vi "Main.vi"(0 "A":dbl=5.0, 5 "B":dbl=7.0, 7 "Calculate":bool, 11 "error in":errorcluster, 13 "Operations":T1) -> (4 "C":dbl, 15 "error out":errorcluster)   [LabVIEW 2023]
doc: "This is a simple calculator which can perform basic arithmetic operations like add, subtract, multiply and divide."
uses:
  Typedef/Operations.ctl
  Typedef/ClassClusters.ctl
  Arithmetic/Arithmetic.lvclass
  Typedef/QueueOperations.ctl
  Children/Multiply/Multiply.lvclass
  Children/Add/Add.lvclass
  Children/Divide/Divide.lvclass
panel:
  # "CALCULATOR"
  # "DISPLAY"
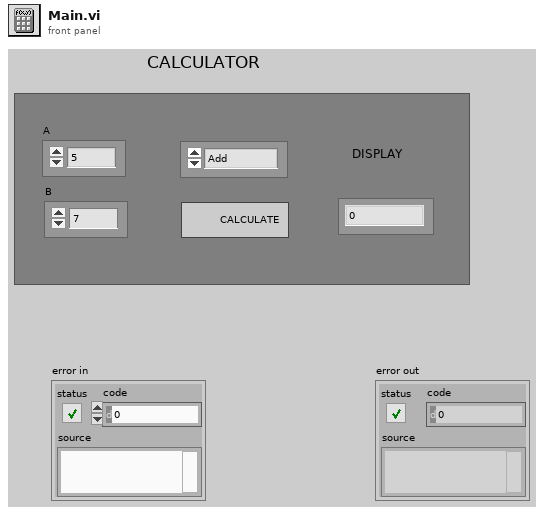
[diagram p1: front panel]
types:
  T1 = typedef "Operations.ctl" = enum16{"Add", "Subtract", "Multiply", "Divide"}
  T2 = typedef "QueueOperations.ctl" = enum16{"Create", "Enqueue", "Enqueue N elements", "Dequeue", "Flush", "Release"}
  T3 = typedef "ClassClusters.ctl" = cluster{"A":dbl, "B":dbl, "C":dbl, "generic class reference":refnum<class "Arithmetic.lvclass">, "Check":bool, "Operations":T1, "Parent Class":refnum<class "Arithmetic.lvclass">, "Add ":refnum<class "Arithmetic.lvclass">, "Subtract":refnum<class "Arithmetic.lvclass">, "Multiply":refnum<class "Arithmetic.lvclass">, "Divide":refnum<class "Arithmetic.lvclass">}
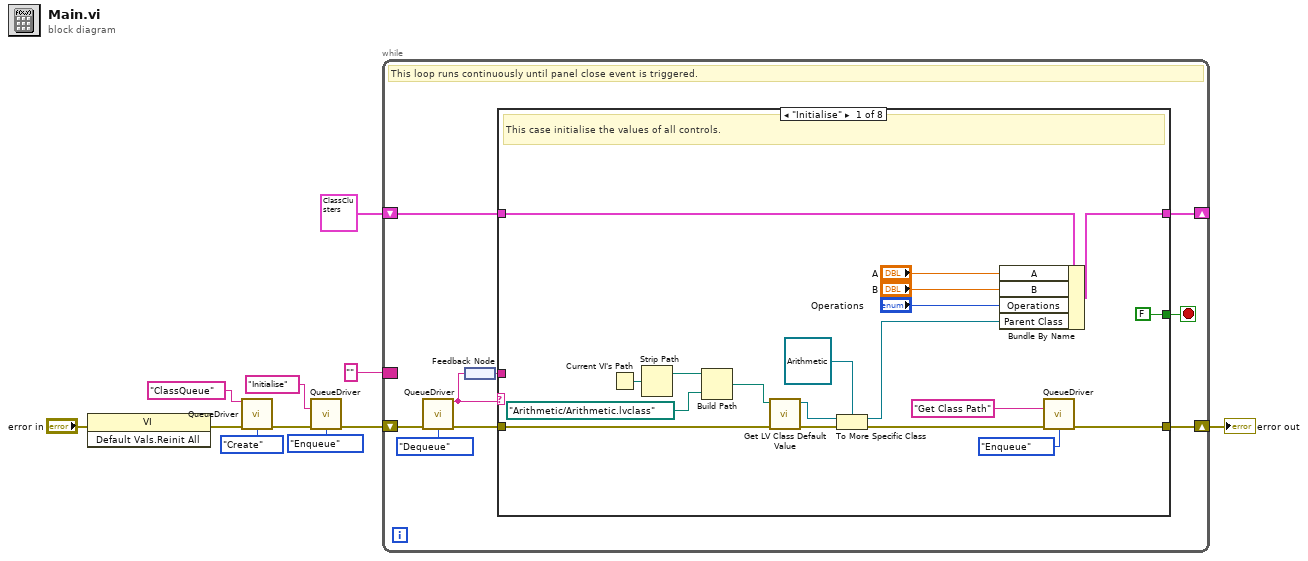
[diagram p0: block diagram]
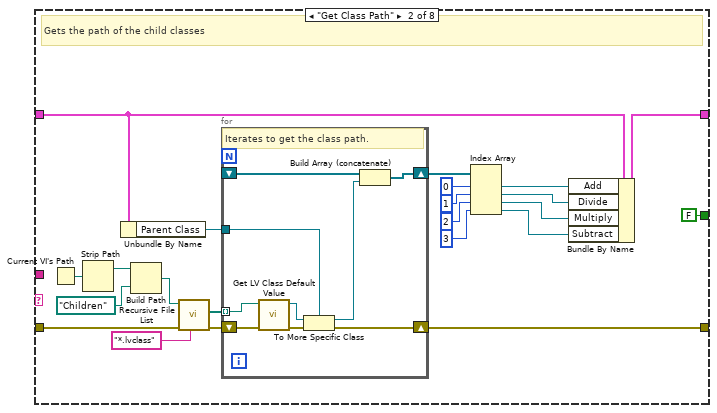
[diagram p2: hidden frame]
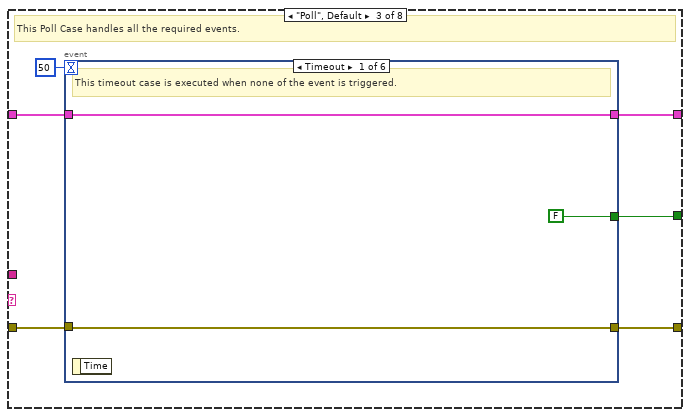
[diagram p3: hidden frame]
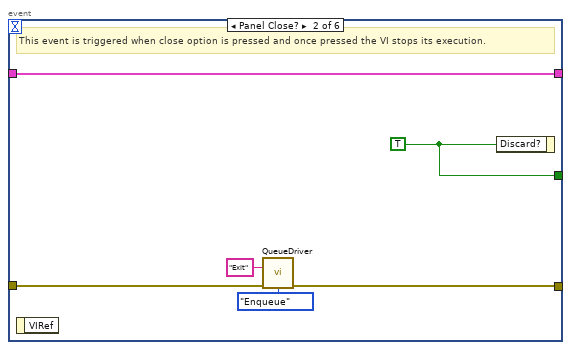
[diagram p4: hidden frame]
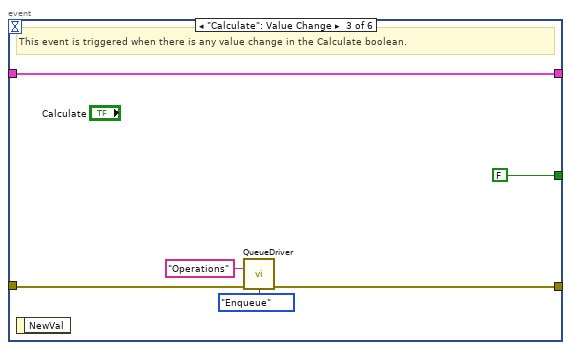
[diagram p5: hidden frame]
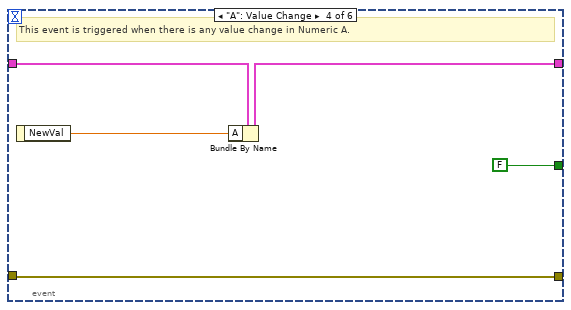
[diagram p6: hidden frame]
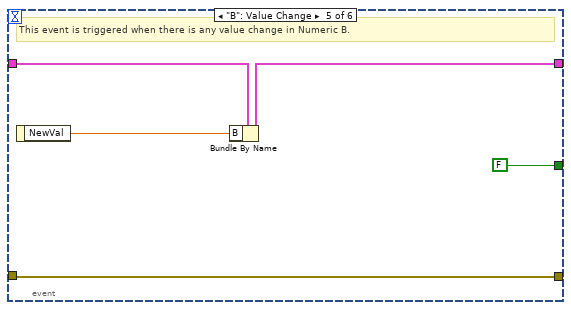
[diagram p7: hidden frame]
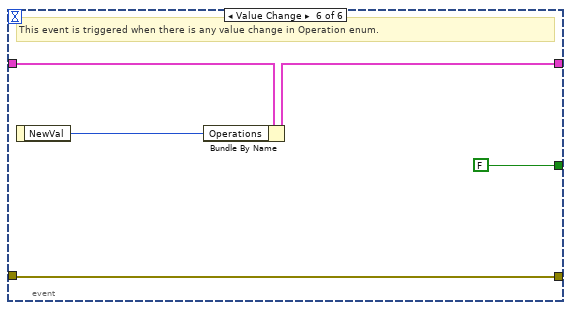
[diagram p8: hidden frame]
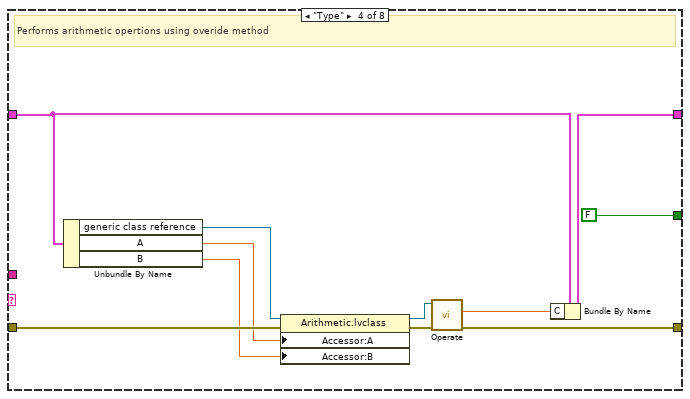
[diagram p9: hidden frame]
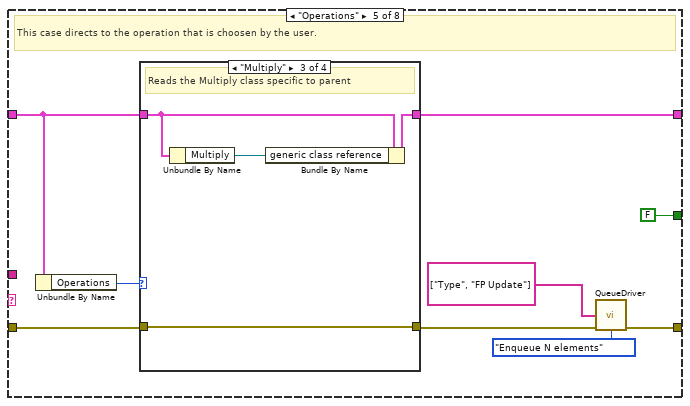
[diagram p10: hidden frame]
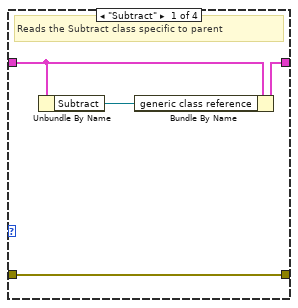
[diagram p11: hidden frame]
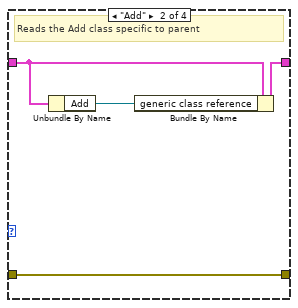
[diagram p12: hidden frame]
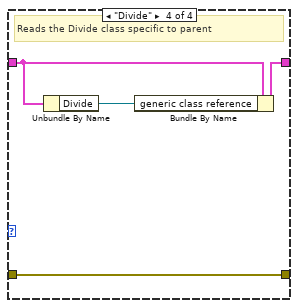
[diagram p13: hidden frame]
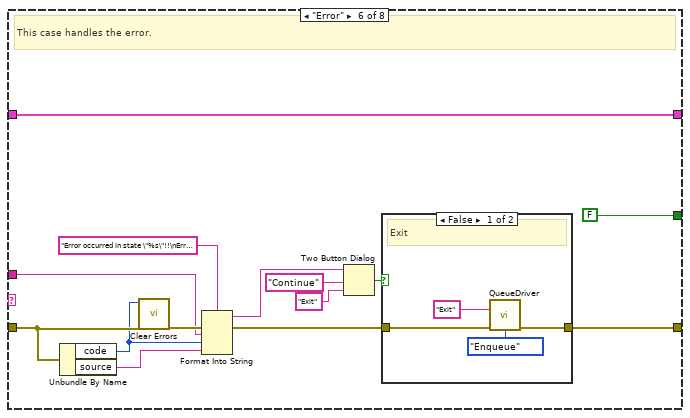
[diagram p14: hidden frame]
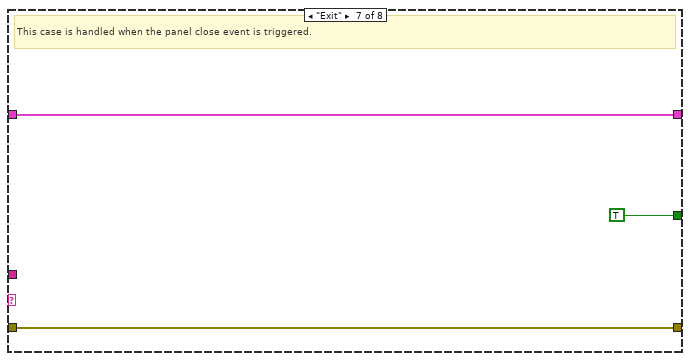
[diagram p16: hidden frame]
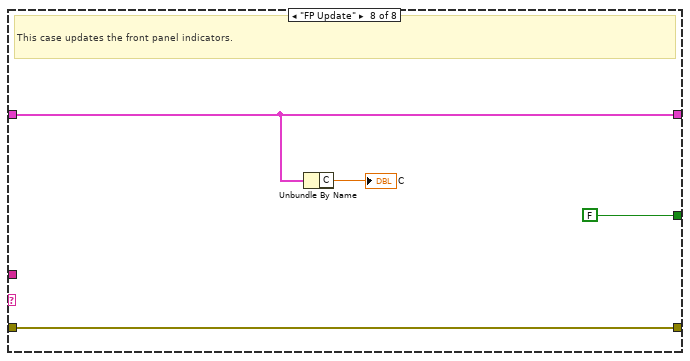
[diagram p17: hidden frame]
diagram:
  n1 = invoke class="VI" method="Default Vals.Reinit All"(error in="error in") -> (error out=w1:errorcluster)  [unwired: 2 in, 2 out]
  n2 = call "QueueDriver.vi"("Queue Name"="ClassQueue", "error in"=w1, "Queue Operations"=QueueOperations."Create") -> ("error out"=w10:errorcluster)  [unwired: 11 in, 1 out]
  n3 = call "QueueDriver.vi"("Enqueue State"="Initialise", "error in"=w10, "Queue Operations"=QueueOperations."Enqueue") -> ("error out"=w9:errorcluster)  [unwired: 11 in, 1 out]
  n4 = while {
    shift-right: [w19] -> _
    shift-left: T3 {"A"=0.0, "B"=0.0, "C"=0.0, "generic class reference"=refnum, "Check"=FALSE, "Operations"=enum."Add", "Parent Class"=refnum, "Add "=refnum, "Subtract"=refnum, "Multiply"=refnum, "Divide"=refnum} -> [w20]
    shift-right: [w15] -> w2
    shift-left: w9 -> [w18]
    border: "" ("Dequeue State") -> [_]
    stop <- w12 stop-if-true
    # "This loop runs continuously until panel close event is triggered."
    n5 = call "QueueDriver.vi"("error in"=w18, "Queue Operations"=QueueOperations."Dequeue") -> ("Dequeue State"=w14:string, "error out"=w17:errorcluster)  [unwired: 12 in]
    n6 = feedback-in #1(w14) -> ()
    n7 = feedback #1() -> (w13:string)
    n8 = case shown="\"Initialise\"" w14 {
      tunnel: w20 -> [w39 w41 w76 w117 w119 w156 w163 w167]
      tunnel: [w38 w46 w75 w110 w118 w156 w163 w167] -> w19
      tunnel: w17 -> [w33 w61 w72 w115 w125 w146 w164 w168]
      tunnel: [w22 w60 w74 w108 w122 w147 w164 w168] -> w15
      tunnel: w13 -> [_ _ _ _ _ w145 _ _]
      tunnel: [FALSE ("Check") FALSE ("Check") w71 FALSE ("Check") FALSE ("Check") FALSE ("Check") TRUE ("Check") FALSE ("Check")] -> w12
      frame "Initialise" {
        # "This case initialise the values of all controls."
        n9 = Current VI's Path() -> (path=w31:path)
        n10 = Strip Path(path=w31) -> (stripped path=w30:path)  [unwired: 1 out]
        n11 = Build Path(base path=w30, name or relative path=path "Arithmetic/Arithmetic.lvclass") -> (appended path=w28:path)
        n12 = call <vilib>:"Get LV Class Default Value.vi"("error in (no error)"=w33, "class path"=w28) -> ("error out"=w32:errorcluster, "object"=w27:refnum<class>)  [unwired: 8 in]
        n13 = To More Specific Class(target class=refnum<class "Arithmetic.lvclass"> refnum ("Arithmetic.lvclass"), reference=w27, error in=w32) -> (specific class reference=w25:refnum<class "Arithmetic.lvclass">, error out=w23:errorcluster)
        n14 = Bundle By Name(cluster=w39, "A"="A", "B"="B", "Operations"="Operations", "Parent Class"=w25) -> (w38:T3)
        n15 = call "QueueDriver.vi"("Enqueue State"="Get Class Path", "error in"=w23, "Queue Operations"=QueueOperations."Enqueue") -> ("error out"=w22:errorcluster)  [unwired: 11 in, 1 out]
      }
      frame "Get Class Path" {
        # "Gets the path of the child classes"
        n16 = Current VI's Path() -> (path=w58:path)
        n17 = Strip Path(path=w58) -> (stripped path=w57:path)  [unwired: 1 out]
        n18 = Unbundle By Name(w41) -> ("Parent Class"=w40:refnum<class "Arithmetic.lvclass">)
        n19 = Build Path(base path=w57, name or relative path=path "Children") -> (appended path=w54:path)
        n20 = call <vilib>:"Recursive File List.vi"("pattern"="*.lvclass", "error in (no error)"=w61, "Folder Path"=w54) -> ("error out"=w55:errorcluster, "All Files in Dir"=w52:path[])  [unwired: 4 in, 3 out]
        n21 = for {
          shift-right: [w65] -> w60
          shift-left: w55 -> [w70]
          shift-right: [w67] -> w51
          shift-left: _ -> [w66]
          tunnel: w52 -> [w69] mode=indexing
          tunnel: w40 -> [w62]
          # "Iterates to get the class path."
          n22 = call <vilib>:"Get LV Class Default Value.vi"("error in (no error)"=w70, "class path"=w69) -> ("error out"=w68:errorcluster, "object"=w64:refnum<class>)  [unwired: 8 in]
          n23 = To More Specific Class(target class=w62, reference=w64, error in=w68) -> (specific class reference=w63:refnum<class "Arithmetic.lvclass">, error out=w65:errorcluster)
          n24 = Build Array (concatenate)(w66, w63) -> (w67:refnum<class "Arithmetic.lvclass">[])
        }
        n25 = Index Array(array=w51, index #1=0 ("index"), index #2=1 ("index"), index #3=2 ("index"), index #4=3 ("index")) -> (element #1=w45:refnum<class "Arithmetic.lvclass">, element #2=w44:refnum<class "Arithmetic.lvclass">, element #3=w43:refnum<class "Arithmetic.lvclass">, element #4=w42:refnum<class "Arithmetic.lvclass">)
        n26 = Bundle By Name(cluster=w41, "Add"=w45, "Divide"=w44, "Multiply"=w43, "Subtract"=w42) -> (w46:T3)
      }
      frame "Poll", Default {
        # "This Poll Case handles all the required events."
        n27 = event shown="[0] Timeout" {
          selector: _ -> [_ _ _ _ _ _]
          dyn-events: _ -> [_ _ _ _ _ _]
          timeout: 50 -> [_ _ _ _ _ _]
          tunnel: w76 -> [w79 w85 w91 w96 w101 w106]
          tunnel: [w79 w85 w91 w94 w99 w104] -> w75
          tunnel: w72 -> [w78 w83 w88 w95 w100 w105]
          tunnel: [w78 w82 w87 w95 w100 w105] -> w74
          tunnel: [FALSE ("Check") w80 FALSE ("Check") FALSE ("Check") FALSE ("Check") FALSE ("Check")] -> w71
          event Timeout {
            # "This timeout case is executed when none of the event is triggered."
            n28 = event-data() -> ()  [unwired: 1 in, 1 out]
          }
          event Panel Close? {
            w80 = TRUE ("Discard?")
            # "This event is triggered when close option is pressed and once pressed the VI stops its execution."
            n29 = event-data() -> ()  [unwired: 1 in, 1 out]
            n30 = call "QueueDriver.vi"("Enqueue State"="Exit", "error in"=w83, "Queue Operations"=QueueOperations."Enqueue") -> ("error out"=w82:errorcluster)  [unwired: 11 in, 1 out]
            n31 = event-data("Discard?"=w80) -> ()  [unwired: 1 in, 1 out]
          }
          event "Calculate": Value Change {
            # "This event is triggered when there is any value change in the Calculate boolean."
            n32 = event-data() -> ()  [unwired: 1 in, 1 out]
            n33 = call "QueueDriver.vi"("Enqueue State"="Operations", "error in"=w88, "Queue Operations"=QueueOperations."Enqueue") -> ("error out"=w87:errorcluster)  [unwired: 11 in, 1 out]
          }
          event "A": Value Change {
            # "This event is triggered when there is any value change in Numeric A."
            n34 = event-data() -> ("NewVal"=w93:dbl)  [unwired: 1 in]
            n35 = Bundle By Name(cluster=w96, "A"=w93) -> (w94:T3)
          }
          event "B": Value Change {
            # "This event is triggered when there is any value change in Numeric B."
            n36 = event-data() -> ("NewVal"=w98:dbl)  [unwired: 1 in]
            n37 = Bundle By Name(cluster=w101, "B"=w98) -> (w99:T3)
          }
          event Value Change {
            # "This event is triggered when there is any value change in Operation enum."
            n38 = event-data() -> ("NewVal"=w103:T1)  [unwired: 1 in]
            n39 = Bundle By Name(cluster=w106, "Operations"=w103) -> (w104:T3)
          }
        }
      }
      frame "Type" {
        # "Performs arithmetic opertions using overide method"
        n40 = Unbundle By Name(w117) -> ("generic class reference"=w116:refnum<class "Arithmetic.lvclass">, "A"=w114:dbl, "B"=w113:dbl)
        n41 = property class="Arithmetic.lvclass"(reference=w116, error in=w115, "Accessor:A"=w114, "Accessor:B"=w113) -> (reference out=w112:refnum<class "Arithmetic.lvclass">, error out=w111:errorcluster)
        n42 = call-dynamic "Operate.vi"("error in (no error)"=w111, "Arithmetic in"=w112) -> ("error out"=w108:errorcluster, "C"=w109:dbl)  [unwired: 7 in, 1 out]
        n43 = Bundle By Name(cluster=w117, "C"=w109) -> (w110:T3)
      }
      frame "Operations" {
        # "This case directs to the operation that is choosen by the user."
        n44 = Unbundle By Name(w119) -> ("Operations"=w126:T1)
        n45 = case shown="\"Multiply\"" w126 {
          tunnel: w125 -> [w130 w134 w138 w142]
          tunnel: [w130 w134 w138 w142] -> w123
          tunnel: w119 -> [w129 w133 w137 w141]
          tunnel: [w128 w132 w136 w140] -> w118
          frame "Subtract" {
            # "Reads the Subtract class specific to parent"
            n46 = Unbundle By Name(w129) -> ("Subtract"=w127:refnum<class "Arithmetic.lvclass">)
            n47 = Bundle By Name(cluster=w129, "generic class reference"=w127) -> (w128:T3)
          }
          frame "Add" {
            # "Reads the Add class specific to parent"
            n48 = Unbundle By Name(w133) -> ("Add"=w131:refnum<class "Arithmetic.lvclass">)
            n49 = Bundle By Name(cluster=w133, "generic class reference"=w131) -> (w132:T3)
          }
          frame "Multiply" {
            # "Reads the Multiply class specific to parent"
            n50 = Unbundle By Name(w137) -> ("Multiply"=w135:refnum<class "Arithmetic.lvclass">)
            n51 = Bundle By Name(cluster=w137, "generic class reference"=w135) -> (w136:T3)
          }
          frame "Divide" {
            # "Reads the Divide class specific to parent"
            n52 = Unbundle By Name(w141) -> ("Divide"=w139:refnum<class "Arithmetic.lvclass">)
            n53 = Bundle By Name(cluster=w141, "generic class reference"=w139) -> (w140:T3)
          }
        }
        n54 = call "QueueDriver.vi"("Array State"=string[] ["Type", "FP Update"], "error in"=w123, "Queue Operations"=QueueOperations."Enqueue N elements") -> ("error out"=w122:errorcluster)  [unwired: 11 in, 1 out]
      }
      frame "Error" {
        # "This case handles the error."
        n55 = Unbundle By Name(w146) -> ("code"=w144:i32, "source"=w148:string)
        n56 = call <vilib>:"Clear Errors.vi"("error in (no error)"=w146, "specific error code to clear (0: all)"=w144) -> ("error out"=w152:errorcluster)  [unwired: 4 in, 1 out]
        n57 = Format Into String(format string="Error occurred in state \"%s\"!!\nError Code: %d\nError Source: %s\n\nDo you wish to continue?", error in=w152, w145, w144, w148) -> (resulting string=w153:string, error out=w155:errorcluster)  [unwired: 1 in]
        n58 = Two Button Dialog(message=w153, 1:"Exit" ("F button name (\"Cancel\")"), 2:"Continue" ("T button name (\"OK\")")) -> (T button?=w154:bool)
        n59 = case shown="False" w154 {
          tunnel: w155 -> [w158 w161]
          tunnel: [w157 w161] -> w147
          frame False {
            # "Exit"
            n60 = call "QueueDriver.vi"("Enqueue State"="Exit", "error in"=w158, "Queue Operations"=QueueOperations."Enqueue") -> ("error out"=w157:errorcluster)  [unwired: 11 in, 1 out]
          }
          frame True {
            # "Continue"
          }
        }
      }
      frame "Exit" {
        # "This case is handled when the panel close event is triggered."
      }
      frame "FP Update" {
        # "This case updates the front panel indicators."
        n61 = Unbundle By Name(w167) -> ("C"=→"C":dbl)
      }
    }
  }
  "error out" <- w2
